vi "Instantiate IntelliSenseString.vi"(5 "Suggestion IO in":refnum<class "SuggestionIObase.lvclass">, 7 "Str Ctl Refnum":refnum<vi>, 9 "Str ctrl Suggestion":string[](array[string]), 11 "error in (no error)":errorcluster) -> (4 "IntelliSense String":refnum<class "IntelliSenseStringControl.lvclass">, 15 "error out":errorcluster)   [LabVIEW 2016, in "StringIntelliSense.lvlib"]
uses:
  StringIntelliSense.lvlib
  Suggestions IO/base/SuggestionIObase.lvclass
  IntelliSenseStringControl.lvclass
  IntelliSenseStringControl.lvclass/IntelliSenseStringControl.ctl
  Private/StringMonitorUserData.vi
  Properties/Set Suggestion List.vi
  Properties/Set Case Sensitive.vi
  Properties/Set String Value Suggestion.vi
  Properties/Set Autofill Suggestion.vi
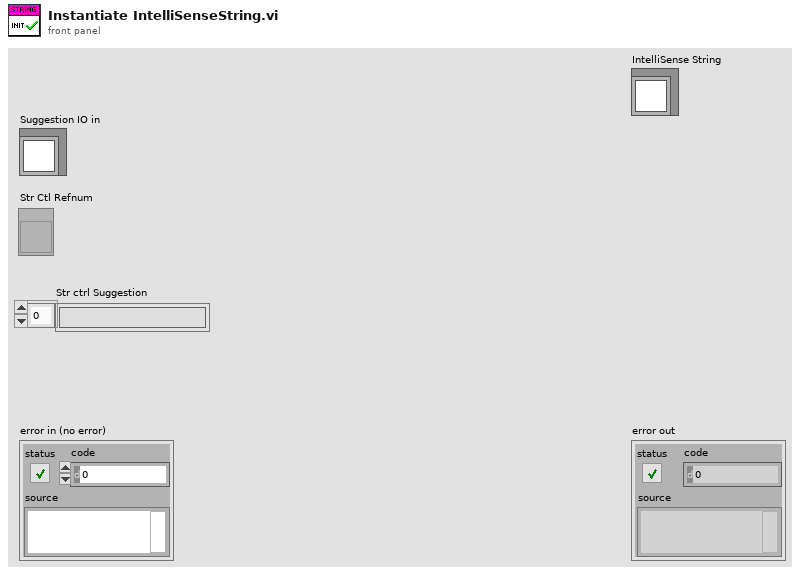
[diagram p1: front panel]
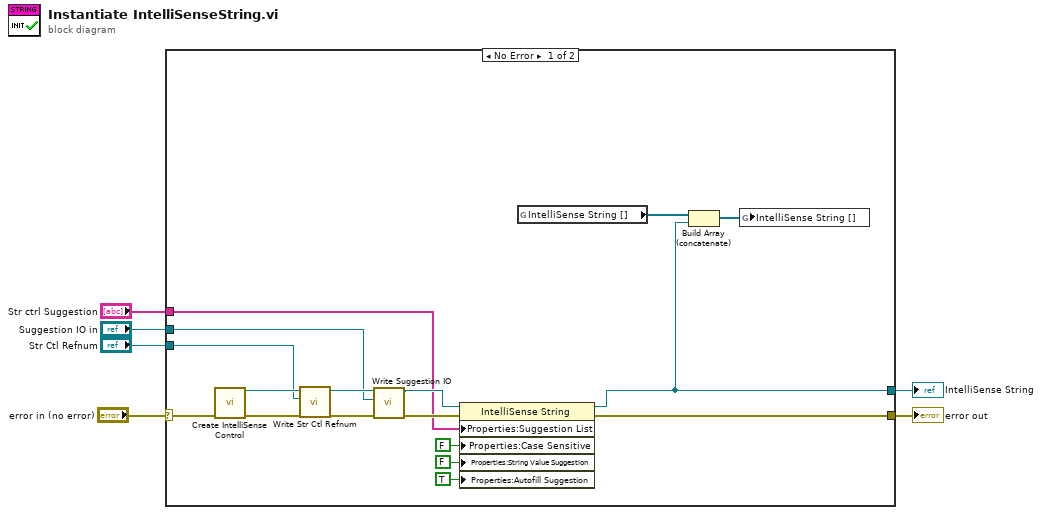
[diagram p0: block diagram]
diagram:
  n1 = case shown="No Error" "error in (no error)" {
    selector: "error in (no error)" -> [w23 w24]
    tunnel: [w12 w24] -> w5
    tunnel: "Suggestion IO in" -> [w15 _]
    tunnel: "Str Ctl Refnum" -> [w16 _]
    tunnel: "Str ctrl Suggestion" -> [w10 _]
    tunnel: [w11 _] -> w1
    frame No Error {
      n2 = call "Create IntelliSense Control.vi"("error in"=w23) -> ("IntelliSense Control"=w20:refnum<class "IntelliSenseStringControl.lvclass">, "error out"=w19:errorcluster)  [unwired: 13 in]
      n3 = call "Write Str Ctl Refnum.vi"("error in (no error)"=w19, "Str Ctl Refnum"=w16, "IntelliSenseStringControl in"=w20) -> ("error out"=w17:errorcluster, "IntelliSenseStringControl out"=w18:refnum<class "IntelliSenseStringControl.lvclass">)  [unwired: 7 in]
      n4 = call "Write Suggestion IO.vi"("error in (no error)"=w17, "Suggestion IO"=w15, "IntelliSenseStringControl in"=w18) -> ("error out"=w14:errorcluster, "IntelliSenseStringControl out"=w13:refnum<class "IntelliSenseStringControl.lvclass">)  [unwired: 7 in]
      n5 = property class="IntelliSense String"(reference=w13, error in=w14, "Properties:Suggestion List"=w10, "Properties:Case Sensitive"=FALSE ("Case Sensitive"), "Properties:String Value Suggestion"=FALSE ("String Value Suggestion"), "Properties:Autofill Suggestion"=TRUE ("Autofill Suggestion")) -> (reference out=w11:refnum<class "IntelliSenseStringControl.lvclass">, error out=w12:errorcluster)
      n6 = global read "StringMonitorUserData.vi" "IntelliSense String []"() -> (w21:refnum<class "IntelliSenseStringControl.lvclass">[])
      n7 = Build Array (concatenate)(w21, w11) -> (w22:refnum<class "IntelliSenseStringControl.lvclass">[])
      n8 = global write "StringMonitorUserData.vi" "IntelliSense String []"(w22) -> ()
    }
    frame Error {
    }
  }
  "error out" <- w5
  "IntelliSense String" <- w1
